vi "Drive Get.vi"(1 "Y":dbl, 2 "X":dbl) -> ()   [LabVIEW 2013]
uses:
  Drive Global Data.vi
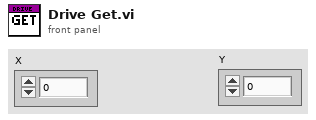
[diagram p1: front panel]
types:
  T1 = cluster{"Y":dbl, "X":dbl, "Left Encoder":dbl, "Right Encoder":dbl}
  T2 = typedef "WPI_EncoderDevRef.ctl" = cluster{"DevStatus":errorcluster, "EncoderIndex":T3, "CounterIndex":T4, "DistancePerCount":dbl, "Decoding Type":T5}
  T3 = typedef "FPGA_EncoderIdx.ctl" = enum8{"Enc 0", "Enc 1", "Enc 2", "Enc 3", "Invalid"}
  T4 = typedef "FPGA_CounterCtrSystemIndex.ctl" = enum8{"Ctr 0", "Ctr 1", "Ctr 2", "Ctr 3", "Ctr 4", "Ctr 5", "Ctr 6", "Ctr 7", "Invalid"}
  T5 = typedef "WPI_EncoderType.ctl" = enum16{"1x", "2x", "4x"}
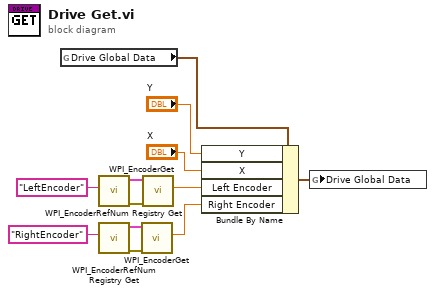
[diagram p0: block diagram]
diagram:
  n1 = global read "Drive Global Data.vi" "Drive Global Data"() -> (w5:T1)
  n2 = call <vilib>:"WPI_EncoderRefNum Registry Get.vi"("refnum name"="LeftEncoder") -> ("error out"=w10:errorcluster, "EncoderDevRef"=w1:T2)  [unwired: 9 in]
  n3 = call <vilib>:"WPI_EncoderRefNum Registry Get.vi"("refnum name"="RightEncoder") -> ("error out"=w8:errorcluster, "EncoderDevRef"=w6:T2)  [unwired: 9 in]
  n4 = call <vilib>:"WPI_EncoderGet.vi"("error in (no error)"=w8, "EncoderDevRef"=w6) -> ("Distance"=w9:dbl)  [unwired: 4 in, 5 out]
  n5 = call <vilib>:"WPI_EncoderGet.vi"("error in (no error)"=w10, "EncoderDevRef"=w1) -> ("Distance"=w12:dbl)  [unwired: 4 in, 5 out]
  n6 = Bundle By Name(cluster=w5, "Y"="Y", "X"="X", "Left Encoder"=w12, "Right Encoder"=w9) -> (w2:T1)
  n7 = global write "Drive Global Data.vi" "Drive Global Data"(w2) -> ()
